vi "DeviceLost.vi"() -> ()   [LabVIEW 2010]
panel:
  in  "stop":bool
  in  "ICImagingControl":refnum<k7>(container)
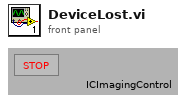
[diagram p1: front panel]
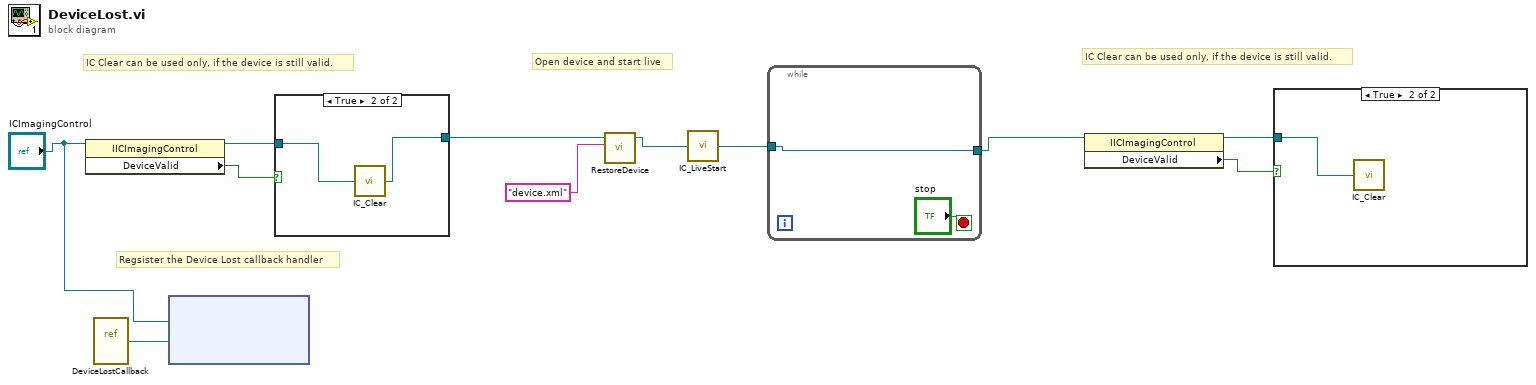
[diagram p0: block diagram]
diagram:
  # "Open device and start live"
  # "Regsister the Device Lost callback handler"
  # "IC Clear can be used only, if the device is still valid."
  # "IC Clear can be used only, if the device is still valid."
  n1 = property class="IICImagingControl"(reference="ICImagingControl") -> (reference out=w5:refnum<k7>, "DeviceValid"=w6:bool)  [unwired: 1 in, 1 out]
  n2 = vi-ref "DeviceLostCallback.vi"() -> ("vi reference"=w10:refnum<vi>)
  n3 = node("ICImagingControl", w10) -> ()  [unwired: 3 in, 2 out]
  n4 = case shown="True" w6 {
    tunnel: w5 -> [w12 w14]
    tunnel: [w12 w13] -> w3
    frame False {
    }
    frame True {
      n5 = call <userlib>:"IC_Clear.vi"("ICImagingControl 2"=w14) -> ("ICImagingControl"=w13:refnum<k7>)
    }
  }
  n6 = call <userlib>:"RestoreDevice.vi"("Filename"="device.xml", "ICImagingControl"=w3) -> ("ICImagingControl 2"=w1:refnum<k7>)  [unwired: 2 in, 2 out]
  n7 = call <userlib>:"IC_LiveStart.vi"("ICImagingControl 3"=w1) -> ("ICImagingControl 2"=w11:refnum<k7>)
  n8 = while {
    tunnel: w11 -> [w15]
    tunnel: [w15] -> w9
    stop <- "stop" stop-if-true
  }
  n9 = property class="IICImagingControl"(reference=w9) -> (reference out=w7:refnum<k7>, "DeviceValid"=w8:bool)  [unwired: 1 in, 1 out]
  n10 = case shown="True" w8 {
    tunnel: w7 -> [_ w17]
    frame False {
    }
    frame True {
      n11 = call <userlib>:"IC_Clear.vi"("ICImagingControl 2"=w17) -> ()  [unwired: 1 out]
    }
  }
